vi "Write Magnetic Deviation Msg.vi"(8 "error in (no error)":errorcluster, 10 "Magnetic Deviation":dbl, 11 "Set Mag Dev Message in":refnum<class "Set Mag Dev Message.lvclass">) -> (0 "error out":errorcluster, 3 "Set Mag Dev Message out":refnum<class "Set Mag Dev Message.lvclass">)   [LabVIEW 2015, in "RDS Child Messages.lvlib" / "Set Mag Dev Message.lvclass"]
uses:
  Set Mag Dev Message.lvclass
  Set Mag Dev Message.lvclass/Set Mag Dev Message.ctl
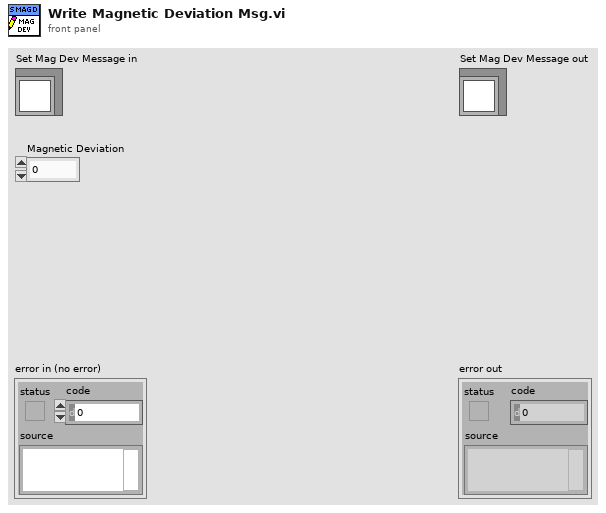
[diagram p1: front panel]
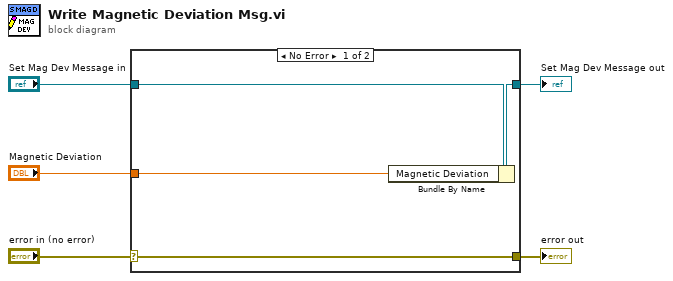
[diagram p0: block diagram]
diagram:
  n1 = case shown="No Error" "error in (no error)" {
    selector: "error in (no error)" -> [w9 w10]
    tunnel: [w9 w10] -> w4
    tunnel: [w7 w11] -> w2
    tunnel: "Set Mag Dev Message in" -> [w8 w11]
    tunnel: "Magnetic Deviation" -> [w6 _]
    frame No Error {
      n2 = Bundle By Name(cluster=w8, "Magnetic Deviation"=w6) -> (w7:refnum<class "Set Mag Dev Message.lvclass">)
    }
    frame Error {
    }
  }
  "error out" <- w4
  "Set Mag Dev Message out" <- w2
